vi "USBData_measure.vi"(0 "USBData in":refnum<class "USBData.lvclass">, 1 "DAQ sample #":i64, 3 "DAQ timeout":dbl, 5 "MeasurementIndex":i64, 11 "error in (no error)":errorcluster) -> (4 "USBData out":refnum<class "USBData.lvclass">, 6 "TimeMeasuremeent":timestamp, 8 "Status":T1(ring), 10 "LastDataAcquired":dbl[](array[numeric]), 12 "Labels":string[](array[string]), 14 "LabelLD":string, 15 "error out":errorcluster)   [LabVIEW 2017, in "USBData.lvclass"]
uses:
  USBData.lvclass
  USBData.lvclass/USBData.ctl
  vi.lib/DAQmx/miscellaneous.llb/DAQmx Fill In Error Info.vi
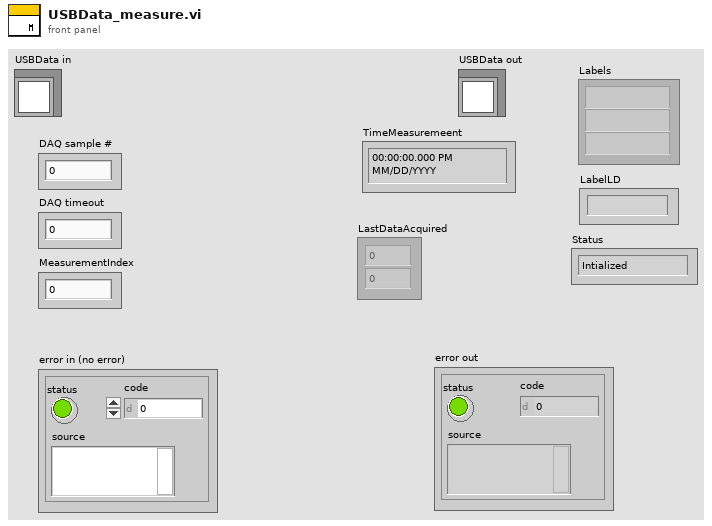
[diagram p1: front panel]
types:
  T1 = enum16{"Intialized", "Waiting", "Measuring", "Terminated"}
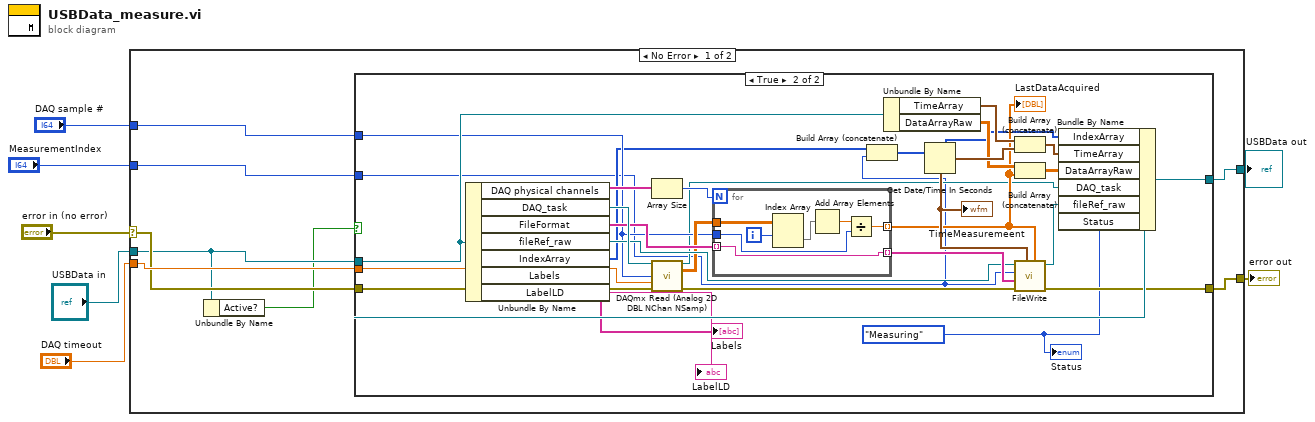
[diagram p0: block diagram]
diagram:
  n1 = case shown="No Error" "error in (no error)" {
    selector: "error in (no error)" -> [w14 w54]
    tunnel: [w11 w54] -> w6
    tunnel: [w13 w53] -> w4
    tunnel: "USBData in" -> [w9 w53]
    tunnel: "DAQ timeout" -> [w15 _]
    tunnel: "DAQ sample #" -> [w10 _]
    tunnel: "MeasurementIndex" -> [w12 _]
    frame No Error {
      n2 = Unbundle By Name(w9) -> ("Active?"=w8:bool)
      n3 = case shown="True" w8 {
        tunnel: w15 -> [_ w45]
        tunnel: w14 -> [w16 w44]
        tunnel: [w17 w40] -> w13
        tunnel: w9 -> [w17 w39]
        tunnel: w12 -> [_ w22]
        tunnel: [w16 w31] -> w11
        tunnel: w10 -> [_ w29]
        frame False {
        }
        frame True {
          w18 = T1."Measuring" ("Status")
          n4 = Unbundle By Name(w39) -> ("DAQ physical channels"=w42:tag[], "DAQ_task"=w43:refnum<k21>, "FileFormat"=w35:string[], "fileRef_raw"=w33:refnum<file>, "IndexArray"=w23:i64[], "Labels"=→"Labels":string[], "LabelLD"=→"LabelLD":string)
          n5 = Array Size(array=w42) -> (size(s)=w41:i32)
          n6 = call "DAQmx Read (Analog 2D DBL NChan NSamp).vi"("task/channels in"=w43, "number of samples per channel"=w29, "timeout"=w45, "error in"=w44) -> ("task out"=w25:refnum<k21>, "data"=w30:dbl[][], "error out"=w32:errorcluster)  [unwired: 9 in]
          n7 = for {
            N: w41 -> [_]
            tunnel: w35 -> [w52] mode=indexing
            tunnel: [w52] -> w34 mode=indexing
            tunnel: w30 -> [w50]
            tunnel: w29 -> [w48]
            tunnel: [w46] -> w27 mode=indexing
            i -> [w51]
            n8 = Index Array(array=w50, index (row)=w51) -> (element=w49:dbl[])  [unwired: 1 in]
            n9 = Add Array Elements(numeric array=w49) -> (sum=w47:dbl)
            n10 = Divide(x=w47, y=w48) -> (x/y=w46:dbl)
          }
          "LastDataAcquired" <- w27
          n11 = Build Array (concatenate)(w23, w22) -> (w21:i64[])
          n12 = Unbundle By Name(w39) -> ("TimeArray"=w38:timestamp[], "DataArrayRaw"=w28:dbl[][])
          n13 = Get Date/Time In Seconds() -> (seconds since 1Jan1904=w36:timestamp)
          "TimeMeasuremeent" <- w36
          n14 = Build Array (concatenate)(w38, w36) -> (w37:timestamp[])
          n15 = Build Array (concatenate)(w28, w27) -> (w26:dbl[][])
          n16 = call "FileWrite.vi"("DataArray"=w27, "Time Stamp"=w36, "Error In"=w32, "FileFormat"=w34, "Index"=w22, "refnum in"=w33) -> ("Error Out"=w31:errorcluster, "Byte Stream File Refnum"=w24:refnum<file>)  [unwired: 4 in]
          n17 = Bundle By Name(cluster=w39, "IndexArray"=w21, "TimeArray"=w37, "DataArrayRaw"=w26, "DAQ_task"=w25, "fileRef_raw"=w24, "Status"=w18) -> (w40:refnum<class "USBData.lvclass">)
          "Status" <- w18
        }
      }
    }
    frame Error {
    }
  }
  "error out" <- w6
  "USBData out" <- w4
